vi "_s_Bronkhorst Serial Auto Setpoints.vi"(7 "Comunicaciones":T3={"Flujo_1"="ASRL6::INSTR", "Brk1"=FALSE, "Flujo_2"="ASRL6::INSTR", "Brk2"=FALSE, "Flujo_3"="ASRL6::INSTR", "Brk3"=FALSE, "Flujo_4"="ASRL6::INSTR", "Brk4"=FALSE, "Eurothe"="ASRL6::INSTR", "Eurot"=FALSE, "Balanza"="ASRL6::INSTR", "Bal"=FALSE, "eValPos"="ASRL6::INSTR", "eVal"=FALSE, "nuVISA"="ASRL6::INSTR", "nu"=FALSE}, 8 "error in (no error)":errorcluster, 11 "Datos":T2 {"Ctrl01" format="%.1f"; "Ctrl03" format="%.1f"; "Ctrl02" format="%.1f"; "Ctrl04" format="%.1f"}) -> (0 "error out":errorcluster, 3 "Setpoints":T1 {"SP4" format="%.2f"; "SP3" format="%.2f"; "SP2" format="%.2f"; "SP1" format="%.2f"})   [LabVIEW 2013]
uses:
  Controles/P2018 Flujos Data.ctl
  Controles/P2019 SetpointsFlows.ctl
  _s_Bronkhorst Control.ctl
panel:
  out "Address":i32
  # "Programando gases"
  # "Auto SP"
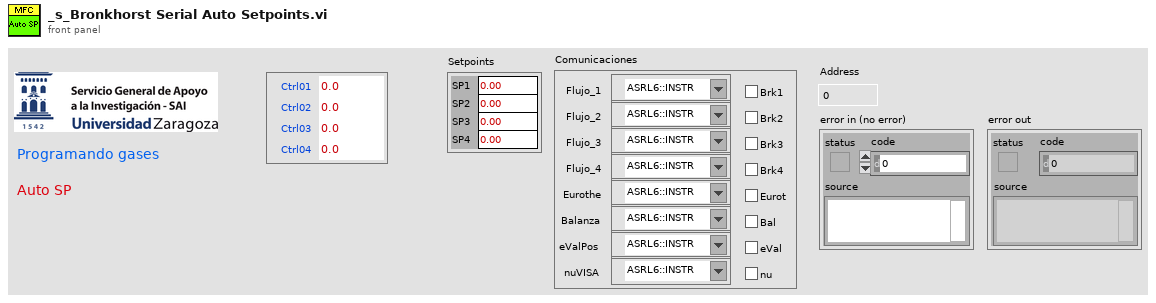
[diagram p1: front panel]
types:
  T1 = typedef "P2019 SetpointsFlows.ctl" = cluster{"SP1":dbl, "SP2":dbl, "SP3":dbl, "SP4":dbl}
  T2 = typedef "P2018 Flujos Data.ctl" = cluster{"Ctrl01":dbl, "Ctrl02":dbl, "Ctrl03":dbl, "Ctrl04":dbl}
  T3 = cluster{"Flujo_1":refnum<visa-resource-name>, "Brk1":bool, "Flujo_2":refnum<visa-resource-name>, "Brk2":bool, "Flujo_3":refnum<visa-resource-name>, "Brk3":bool, "Flujo_4":refnum<visa-resource-name>, "Brk4":bool, "Eurothe":refnum<visa-resource-name>, "Eurot":bool, "Balanza":refnum<visa-resource-name>, "Bal":bool, "eValPos":refnum<visa-resource-name>, "eVal":bool, "nuVISA":refnum<visa-resource-name>, "nu":bool}
  T4 = typedef "_s_Bronkhorst Control.ctl" = enum16{"Inicializar", "Request IdnString", "Request Serial Number", "Request Fluid Number", "Request Fluid Name", "Request Sensor Type", "Request Cap 0", "Request Cap100", "Request Units", "Request CapUnitStr", "Request Setpoint %", "Request Setpoint", "Request Measure %", "Request Measure ", "Send Control Mode", "Send Fluid Number", "Send Setpoint %", "Send Setpoint", "Shutdown"}
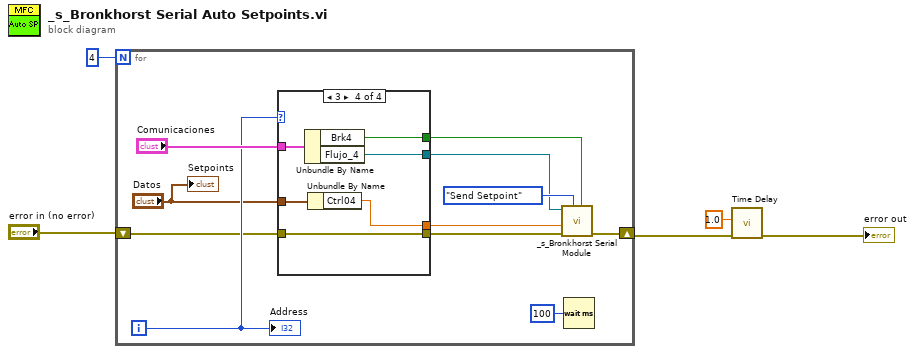
[diagram p0: block diagram]
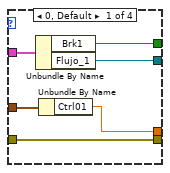
[diagram p2: hidden frame]
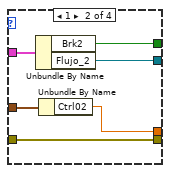
[diagram p3: hidden frame]
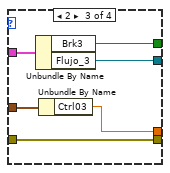
[diagram p4: hidden frame]
diagram:
  n1 = for {
    N: 4 -> [_]
    shift-right: [w10] -> w2
    shift-left: "error in (no error)" -> [w9]
    i -> [w15]
    n2 = case shown="3" w15 {
      tunnel: w9 -> [w20 w26 w32 w38]
      tunnel: "Comunicaciones" -> [w22 w28 w34 w40]
      tunnel: [w21 w27 w33 w39] -> w12
      tunnel: [w20 w26 w32 w38] -> w11
      tunnel: [w19 w25 w31 w37] -> w13
      tunnel: "Datos" -> [w18 w24 w30 w36]
      tunnel: [w17 w23 w29 w35] -> w7
      frame 0, Default {
        n3 = Unbundle By Name(w22) -> ("Brk1"=w21:bool, "Flujo_1"=w19:refnum<visa-resource-name>)
        n4 = Unbundle By Name(w18) -> ("Ctrl01"=w17:dbl)
      }
      frame 1 {
        n5 = Unbundle By Name(w28) -> ("Brk2"=w27:bool, "Flujo_2"=w25:refnum<visa-resource-name>)
        n6 = Unbundle By Name(w24) -> ("Ctrl02"=w23:dbl)
      }
      frame 2 {
        n7 = Unbundle By Name(w34) -> ("Brk3"=w33:bool, "Flujo_3"=w31:refnum<visa-resource-name>)
        n8 = Unbundle By Name(w30) -> ("Ctrl03"=w29:dbl)
      }
      frame 3 {
        n9 = Unbundle By Name(w40) -> ("Brk4"=w39:bool, "Flujo_4"=w37:refnum<visa-resource-name>)
        n10 = Unbundle By Name(w36) -> ("Ctrl04"=w35:dbl)
      }
    }
    n11 = call "_s_Bronkhorst Serial Module.vi"("Module (T:Enable)"=w12, "Command"=_s_Bronkhorst_Control."Send Setpoint", "error in (no error)"=w11, "Setpoint %"=w7, "VISA resource name"=w13) -> ("error out"=w10:errorcluster)  [unwired: 3 in, 3 out]
    n12 = Wait (ms)(milliseconds to wait=u32 100) -> ()  [unwired: 1 out]
    "Address" <- w15
    "Setpoints" <- "Datos"
  }
  n13 = call "Time Delay"("error in (no error)"=w2, "Delay Time (s)"=1.0) -> ("error out"=→"error out":errorcluster)  [unwired: 9 in]
